vi "zmq_recv_timeout.vi"(4 "error in":errorcluster, 5 "timeout (ms)":u32=500, 7 "socket in":refnum<class "Socket.lvclass">) -> (0 "error out":errorcluster, 1 "timeout?":bool, 2 "parts":string[](array[string]), 3 "socket out":refnum<class "Socket.lvclass">)   [LabVIEW 2025, in "ZeroMQ.lvlib" / "Socket.lvclass"]
doc: "An implementation of \"receive with timeout\" functionality, returning an array of strings as per zmq_recv_multi. This VI is provided as a development \"crutch\" and is against the ZeroMQ philosophy but is highly convenient in some situations.\n\nPolls <b>socket in</b> periodically every <b>poll interval</b> milliseconds until a message has been received, or <b>timeout</b> milliseconds elapses since the start of the call. Aborts on error.\n\nDetailed API documentation: http://api.zeromq.org/3-2:zmq-poll"
uses:
  Socket.lvclass
  Socket.lvclass/Socket.ctl
  ZeroMQ.lvlib
panel:
  # "ØMQ"
  # "labview"
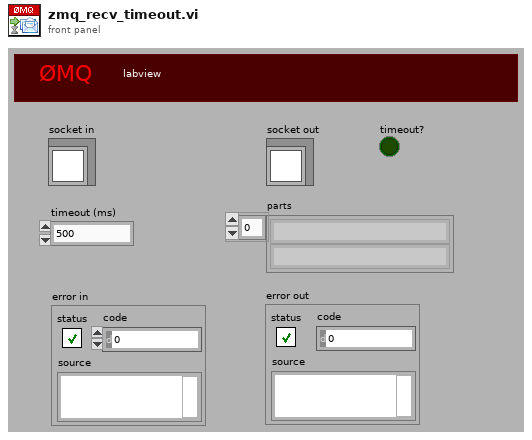
[diagram p1: front panel]
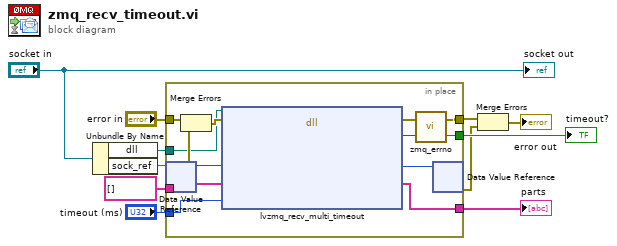
[diagram p0: block diagram]
diagram:
  n1 = Unbundle By Name("socket in") -> ("dll"=w1:path, "sock_ref"=w4:refnum<data-value>)
  n2 = in-place {
    in-place-border: string[] [] ("parts") -> [w24]
    in-place-border: [w23] -> w10
    in-place-border: "timeout (ms)" -> [w22]
    in-place-border: "error in" -> [w21]
    in-place-border: [w18] -> w7
    in-place-border: [w17] -> w6
    in-place-border: w1 -> [w12]
    n3 = in-place-dvr #1(w4) -> (w16:u64, w13:errorcluster)
    n4 = Merge Errors(w21, w13) -> (w14:errorcluster)
    n5 = dll-call lib="?" fn="lvzmq_recv_multi_timeout" ("zmq_labview.dll:lvzmq_socket")(path in=w12, error in=w14, "sock_obj"=w16, "data"=w24, "timeout"=w22) -> (error out=w20:errorcluster, "return type"=w19:i32, "sock_obj"=w15:u64, "data"=w23:string[])  [unwired: 4 in, 1 out]
    n6 = call "zmq_errno.vi"("retval"=w19, "error in"=w20) -> ("again?"=w17:bool, "error out"=w18:errorcluster)
    n7 = in-place-dvr #1(w15) -> (w2:errorcluster)  [unwired: 1 out]
  }
  "parts" <- w10
  "timeout?" <- w6
  n8 = Merge Errors(w7, w2) -> (→"error out":errorcluster)
  "socket out" <- "socket in"
